vi "Abort Measurement.vi"(8 "error in (no error)":errorcluster, 11 "User Interface in":refnum<class "User Interface.lvclass">) -> (0 "error out":errorcluster, 3 "User Interface out":refnum<class "User Interface.lvclass">)   [LabVIEW 2016, in "User Interface.lvlib" / "User Interface.lvclass"]
uses:
  User Interface.lvclass
  <vilib>/ActorFramework/Message Enqueuer/Message Enqueuer.lvclass/Message Enqueuer.ctl
  <vilib>/ActorFramework/Message Enqueuer/Enqueue.vi
  <vilib>/ActorFramework/Stop Msg/Stop Msg.lvclass
  C:/Program Files (x86)/National Instruments/LabVIEW 2016/vi.lib/ActorFramework/Message/Message.lvclass
  <vilib>/ActorFramework/Message Priority Queue/Priority Enqueue.vi
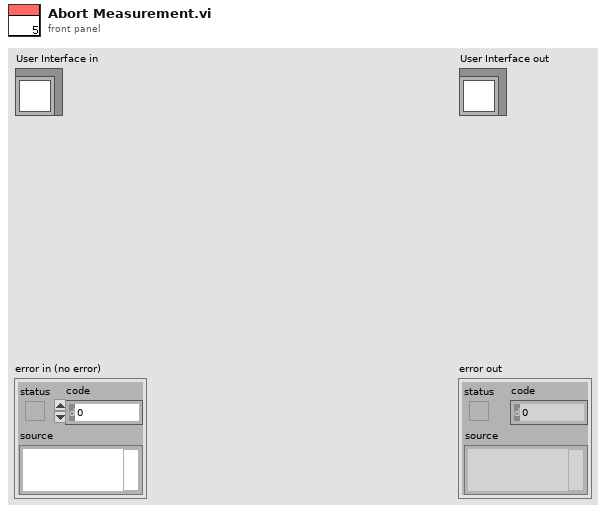
[diagram p1: front panel]
types:
  T1 = enum8{"Enabled", "Disabled", "Disabled and Grayed Out"}
  T2 = typedef "User Interface.lvlib/Buttons.ctl" = cluster{"Start":refnum<vi>, "Save Results":refnum<vi>, "Abort":refnum<vi>, "Hardware Settings":refnum<vi>}
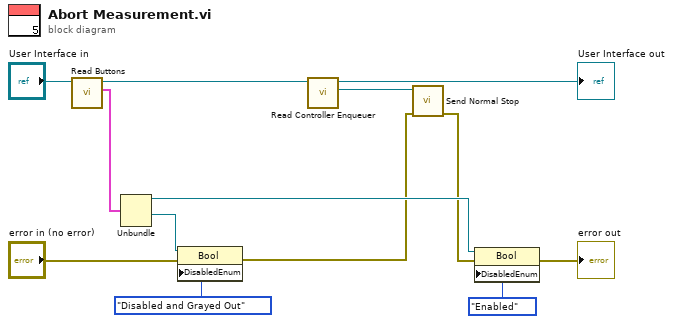
[diagram p0: block diagram]
diagram:
  n1 = call-dynamic "Read Buttons.vi"("User Interface in"="User Interface in") -> ("Buttons"=w12:T2, "User Interface out"=w5:refnum<class "User Interface.lvclass">)  [unwired: 9 in]
  n2 = Unbundle(w12) -> ("Start"=w6:refnum<vi>, "Abort"=w7:refnum<vi>)  [unwired: 2 out]
  n3 = property class="Bool"(reference=w7, error in="error in (no error)", "DisabledEnum"=T1."Disabled and Grayed Out" ("Disabled")) -> (error out=w2:errorcluster)  [unwired: 1 out]
  n4 = call-dynamic "Read Controller Enqueuer.vi"("User Interface in"=w5) -> ("Actor Framework:Message Enqueuer"=w4:refnum<class "Message Enqueuer.lvclass">, "User Interface out"=→"User Interface out":refnum<class "User Interface.lvclass">)  [unwired: 9 in]
  n5 = call <vilib>:"Send Normal Stop.vi"("error in (no error)"=w2, "Message Enqueuer"=w4) -> ("error out"=w1:errorcluster)  [unwired: 9 in]
  n6 = property class="Bool"(reference=w6, error in=w1, "DisabledEnum"=T1."Enabled" ("Disabled")) -> (error out=→"error out":errorcluster)  [unwired: 1 out]
